vi "Boiler Controller.vi"(8 "error in":errorcluster, 9 "Controller Configuration":T1, 10 "Notifiers":T2, 11 "Message Queues":T3) -> (0 "error out":errorcluster)   [LabVIEW 2014, in "Controller.lvlib"]
uses:
  Controller.lvlib
  support/Message Queue/All Message Queues.ctl
  support/Message Queue/Message Cluster.ctl
  support/Notifiers/Notifiers.ctl
  Controller Configuration.ctl
  controls/MHL UI Data.ctl
  controls/MHL Status.ctl
  support/Boiler System Globals.vi
  <vilib>/Utility/error.llb/Error Cluster From Error Code.vi
  <vilib>/ErrorRing/Error Ring.xnode
  support/Message Queue/Message Queue.lvlib
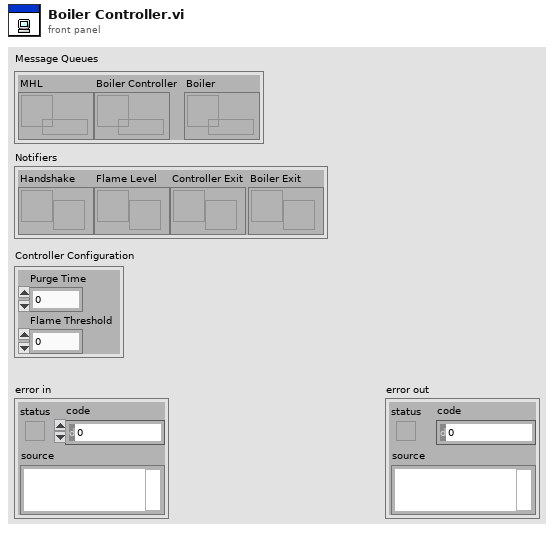
[diagram p1: front panel]
types:
  T1 = typedef "Controller.lvlib/Controller Configuration.ctl" = cluster{"Purge Time":u32, "Flame Threshold":u32}
  T2 = typedef "Notifiers.ctl" = cluster{"Handshake":refnum<notifier>, "Flame Level":refnum<notifier>, "Controller Exit":refnum<notifier>, "Boiler Exit":refnum<notifier>}
  T3 = typedef "Message Queue.lvlib/All Message Queues.ctl" = cluster{"MHL":refnum<queue>, "Boiler Controller":refnum<queue>, "Boiler":refnum<queue>}
  T4 = enum16{"open", "replace", "create", "open or create", "replace or create", "replace or create with confirmation"}
  T5 = typedef "MHL Status.ctl" = enum16{"Lockout", "Ready", "Pre-Purge", "Pre-Purge Complete", "Pilot On", "Boiler Running", "Shutdown", "Purge"}
  T6 = typedef "MHL UI Data.ctl" = cluster{"Status":string, "Fuel Control Valve":u32, "Primary Fan":bool, "Pilot Gas Valve":bool, "Pilot":bool, "Forced Draft Fan":bool, "MHL Status":T5}
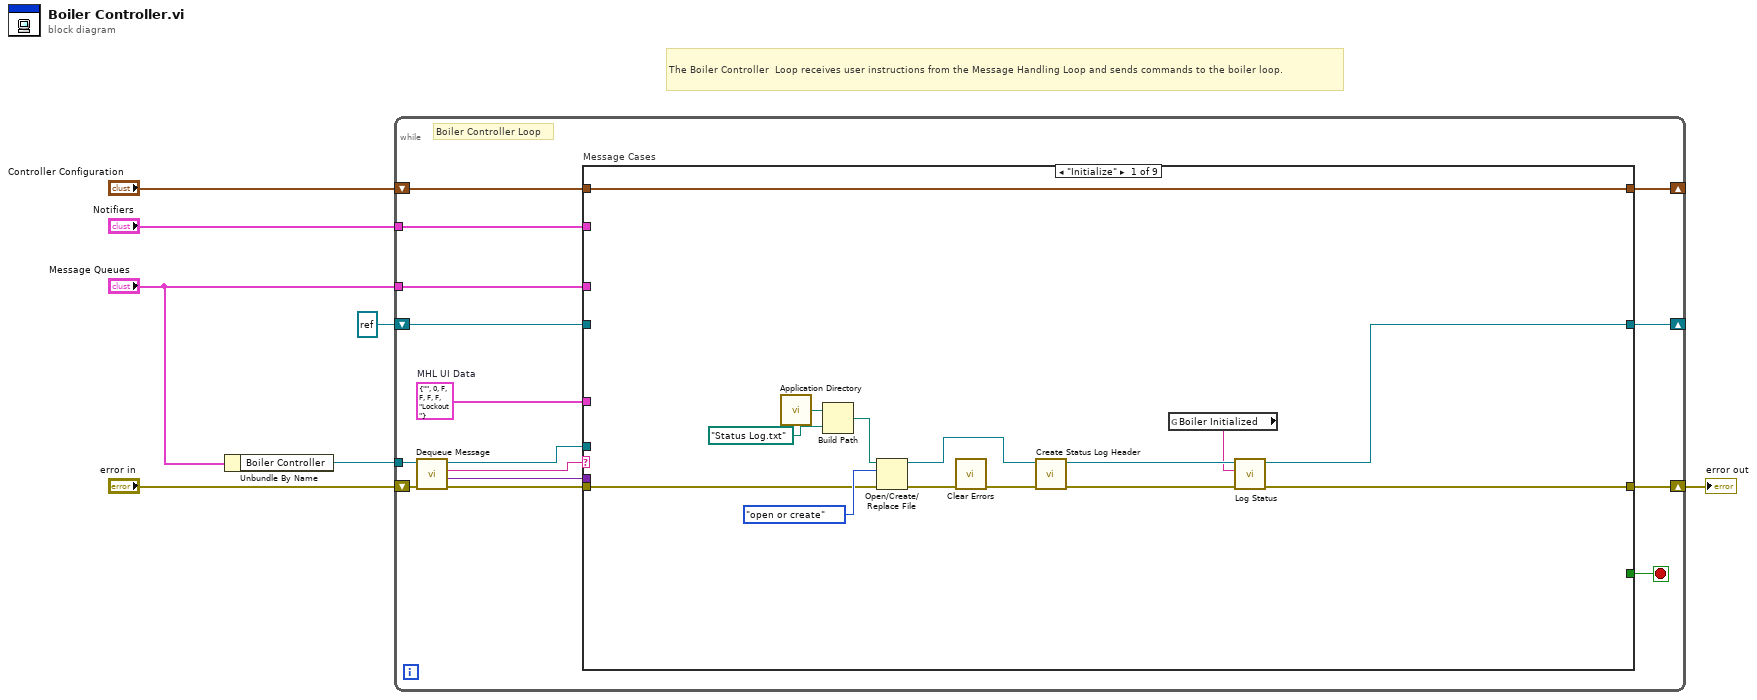
[diagram p0: block diagram]
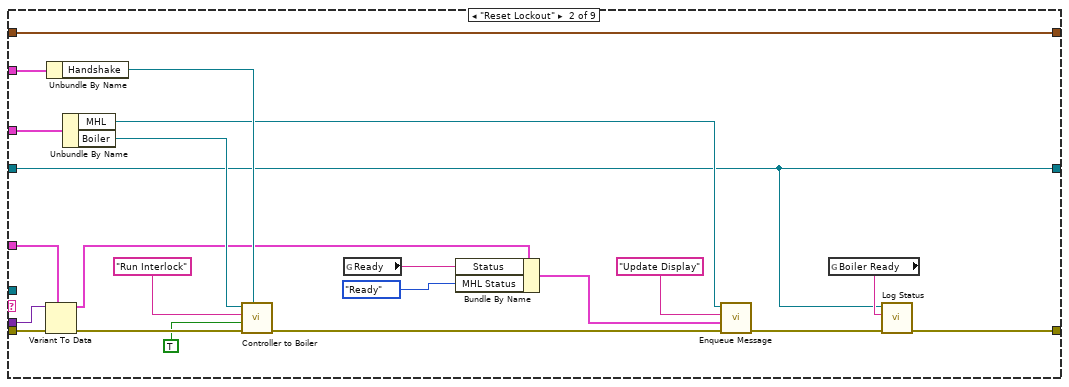
[diagram p2: hidden frame]
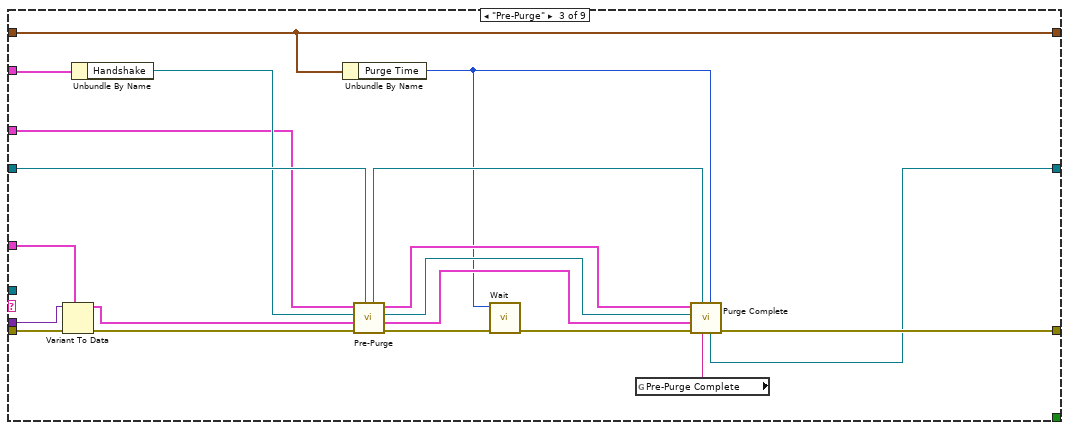
[diagram p3: hidden frame]
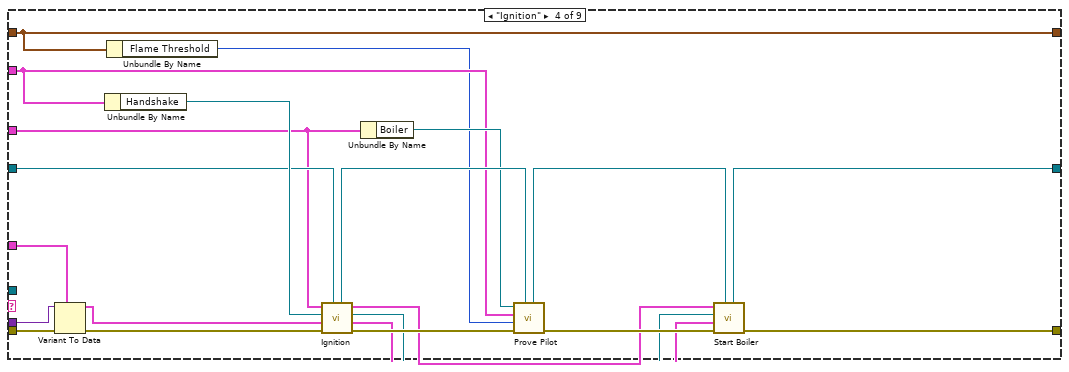
[diagram p4: hidden frame]
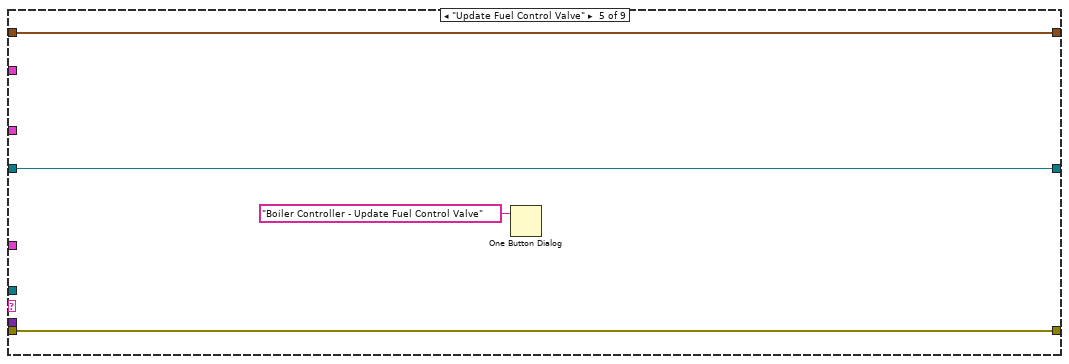
[diagram p5: hidden frame]
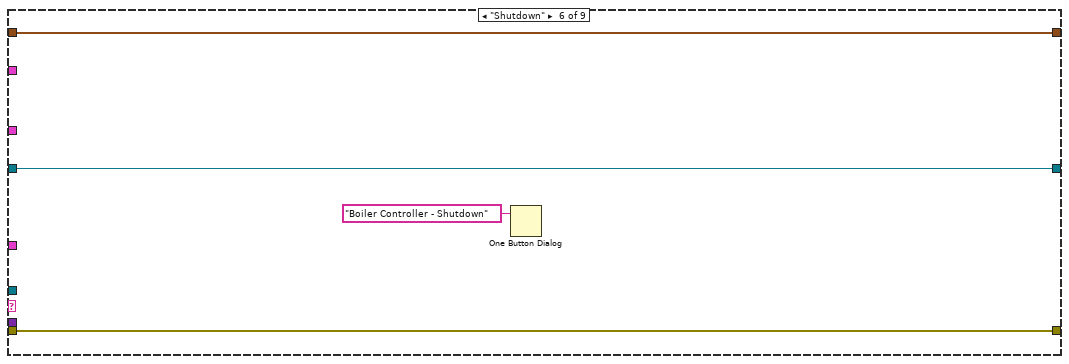
[diagram p6: hidden frame]
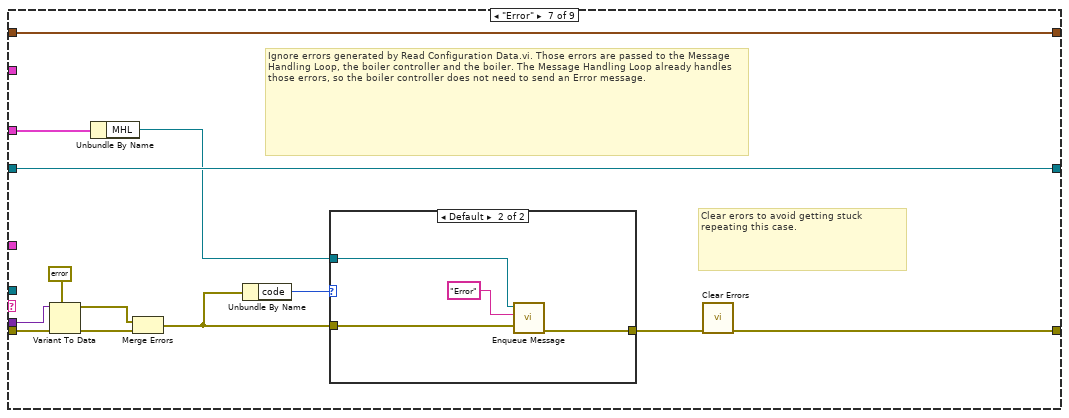
[diagram p7: hidden frame]
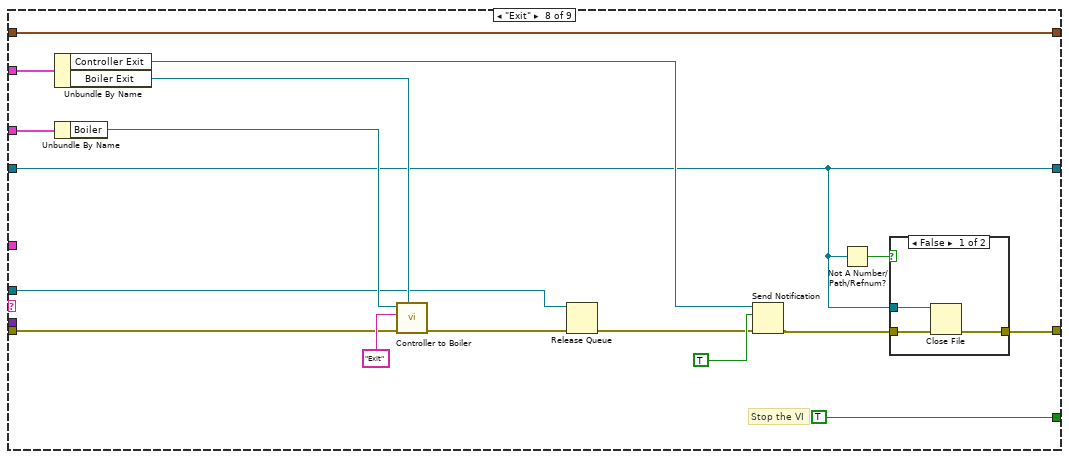
[diagram p9: hidden frame]
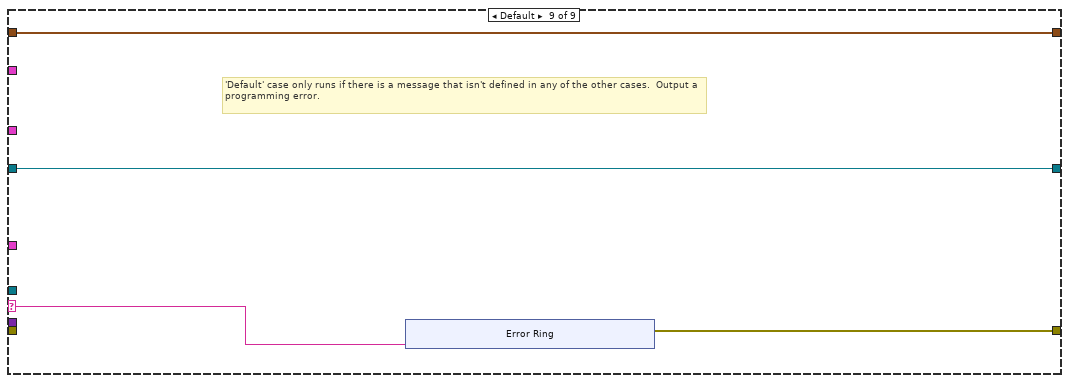
[diagram p11: hidden frame]
diagram:
  # "The Boiler Controller  Loop receives user instructions from the Message Handling Loop and sends commands to the boiler loop."
  n1 = Unbundle By Name("Message Queues") -> ("Boiler Controller"=w5:refnum<queue>)
  n2 = while {
    tunnel: w5 -> [w16]
    shift-right: [w15] -> w7
    shift-left: "error in" -> [w21]
    tunnel: "Message Queues" -> [w14]
    tunnel: "Notifiers" -> [w13]
    shift-right: [w12] -> _
    shift-left: refnum<file> refnum ("Log File Refnum out") -> [w11]
    shift-right: [w9] -> _
    shift-left: "Controller Configuration" -> [w8]
    stop <- w22 stop-if-true
    w10 = T6 {"Status"="", "Fuel Control Valve"=0, "Primary Fan"=FALSE, "Pilot Gas Valve"=FALSE, "Pilot"=FALSE, "Forced Draft Fan"=FALSE, "MHL Status"=enum."Lockout"}  # MHL UI Data
    # "Boiler Controller Loop"
    n3 = call "Dequeue Message.vi"("error in (no error)"=w21, "Message Queue"=w16) -> ("error out"=w20:errorcluster, "Message Data"=w18:variant, "Message"=w19:string, "dup Message Queue"=w17:refnum<queue>)  [unwired: 6 in]
    n4 = case "Message Cases" shown="\"Initialize\"" w19 {
      selector: w19 -> [_ _ _ _ _ _ _ _ w149]
      tunnel: w17 -> [_ _ _ _ _ _ _ w135 _]
      tunnel: w20 -> [w26 w58 w78 w99 w103 w107 w119 w134 _]
      tunnel: [w27 w54 w66 w79 w103 w107 w110 w127 w150] -> w15
      tunnel: [_ _ _ _ _ _ _ TRUE _] -> w22
      tunnel: w18 -> [_ w53 w76 w95 _ _ w117 _ _]
      tunnel: w14 -> [_ w51 w70 w89 _ _ w120 w132 _]
      tunnel: w13 -> [_ w49 w73 w87 _ _ _ w131 _]
      tunnel: [w25 w39 w64 w80 w101 w105 w114 w126 w148] -> w12
      tunnel: w11 -> [_ w39 w72 w91 w101 w105 w114 w126 w148]
      tunnel: w10 -> [_ w52 w75 w94 _ _ _ _ _]
      tunnel: w8 -> [w24 w37 w68 w86 w100 w104 w113 w130 w147]
      tunnel: [w24 w37 w68 w86 w100 w104 w113 w130 w147] -> w9
      frame "Initialize" {
        n5 = call <vilib>:"Application Directory.vi"() -> ("Application Directory"=w29:path)
        n6 = Build Path(base path=w29, name or relative path=path "Status Log.txt") -> (appended path=w33:path)
        n7 = Open/Create/Replace File(file path (use dialog)=w33, error in=w26, operation (0:open)=T4."open or create") -> (refnum out=w30:refnum<file>, error out=w31:errorcluster)  [unwired: 3 in, 1 out]
        n8 = call <vilib>:"Clear Errors.vi"("error in (no error)"=w31) -> ("error out"=w23:errorcluster)  [unwired: 5 in, 1 out]
        n9 = call "Create Status Log Header.vi"("error in"=w23, "Log File Refnum in"=w30) -> ("error out"=w36:errorcluster, "Log File Refnum out"=w35:refnum<file>)  [unwired: 8 in]
        n10 = global read "Boiler System Globals.vi" "Boiler Initialized"() -> (w34:string)
        n11 = call "Log Status.vi"("error in"=w36, "Event String"=w34, "Log File Refnum In"=w35) -> ("error out"=w27:errorcluster, "Log File Refnum Out"=w25:refnum<file>)  [unwired: 7 in]
      }
      frame "Reset Lockout" {
        n12 = Variant To Data(error in=w58, type=w52, Variant=w53) -> (data=w45:T6, error out=w57:errorcluster)
        n13 = Unbundle By Name(w49) -> ("Handshake"=w48:refnum<notifier>)
        n14 = Unbundle By Name(w51) -> ("MHL"=w41:refnum<queue>, "Boiler"=w50:refnum<queue>)
        n15 = call "Controller to Boiler.vi"("Notifier"=w48, "error in"=w57, "Message Data"=TRUE, "Message"="Run Interlock", "Boiler Queue in"=w50) -> ("error out"=w56:errorcluster)  [unwired: 4 in, 2 out]
        n16 = global read "Boiler System Globals.vi" "Ready"() -> (w44:string)
        n17 = Bundle By Name(cluster=w45, "Status"=w44, "MHL Status"=MHL_Status."Ready") -> (w43:T6)
        n18 = call "Enqueue Message.vi"("error in (no error)"=w56, "Message Data"=w43, "Message"="Update Display", "Message Queue"=w41) -> ("error out"=w55:errorcluster)  [unwired: 6 in, 1 out]
        n19 = global read "Boiler System Globals.vi" "Boiler Ready"() -> (w40:string)
        n20 = call "Log Status.vi"("error in"=w55, "Event String"=w40, "Log File Refnum In"=w39) -> ("error out"=w54:errorcluster)  [unwired: 7 in, 1 out]
      }
      frame "Pre-Purge" {
        n21 = Variant To Data(error in=w78, type=w75, Variant=w76) -> (data=w74:T6, error out=w77:errorcluster)
        n22 = Unbundle By Name(w73) -> ("Handshake"=w71:refnum<notifier>)
        n23 = Unbundle By Name(w68) -> ("Purge Time"=w60:u32)
        n24 = call "Pre-Purge.vi"("Log File Refnum in"=w72, "error in"=w77, "UI Data in"=w74, "Handshake Notifier in"=w71, "Message Queues in"=w70) -> ("error out"=w69:errorcluster, "UI Data out"=w63:T6, "Handshake Notifier out"=w62:refnum<notifier>, "Message Queues out"=w61:T3, "Log File Refnum out"=w65:refnum<file>)  [unwired: 2 in]
        n25 = call "Wait.vi"("error in"=w69, "Purge Time (s)"=w60) -> ("error out"=w67:errorcluster)  [unwired: 9 in]
        n26 = global read "Boiler System Globals.vi" "Pre-Purge Complete"() -> (w59:string)
        n27 = call "Purge Complete.vi"("Purge Time"=w60, "Status"=w59, "Log File Refnum in"=w65, "error in"=w67, "UI Data in"=w63, "Handshake Notifier in"=w62, "Message Queues in"=w61) -> ("error out"=w66:errorcluster, "Log File Refnum out"=w64:refnum<file>)  [unwired: 3 out]
      }
      frame "Ignition" {
        n28 = Variant To Data(error in=w99, type=w94, Variant=w95) -> (data=w93:T6, error out=w98:errorcluster)
        n29 = Unbundle By Name(w87) -> ("Handshake"=w92:refnum<notifier>)
        n30 = Unbundle By Name(w86) -> ("Flame Threshold"=w85:u32)
        n31 = call "Ignition.vi"("Log File Refnum in"=w91, "error in"=w98, "UI Data in"=w93, "Handshake Notifier in"=w92, "Message Queues in"=w89) -> ("error out"=w97:errorcluster, "UI Data out"=w84:T6, "Handshake Notifier out"=w83:refnum<notifier>, "Message Queues out"=w82:T3, "Log File Refnum out"=w90:refnum<file>)  [unwired: 2 in]
        n32 = Unbundle By Name(w89) -> ("Boiler"=w88:refnum<queue>)
        n33 = call "Prove Pilot.vi"("Log File Refnum in"=w90, "error in"=w97, "Flame Threshold"=w85, "Notifiers in"=w87, "Boiler Queue in"=w88) -> ("error out"=w96:errorcluster, "Log File Refnum out"=w81:refnum<file>)  [unwired: 3 in, 2 out]
        n34 = call "Start Boiler.vi"("Log File Refnum in"=w81, "error in"=w96, "UI Data in"=w84, "Handshake Notifier in"=w83, "Message Queues in"=w82) -> ("error out"=w79:errorcluster, "Log File Refnum out"=w80:refnum<file>)  [unwired: 2 in, 3 out]
      }
      frame "Update Fuel Control Valve" {
        n35 = One Button Dialog(message="Boiler Controller - Update Fuel Control Valve") -> ()  [unwired: 1 in, 1 out]
      }
      frame "Shutdown" {
        n36 = One Button Dialog(message="Boiler Controller - Shutdown") -> ()  [unwired: 1 in, 1 out]
      }
      frame "Error" {
        # "Ignore errors generated by Read Configuration Data.vi. Those errors are passed to the Message Handling Loop, the boiler controller and the boiler. The Message Handling Loop already handles those errors, so the boiler controller does not need to send an Error message."
        # "Clear erors to avoid getting stuck repeating this case."
        n37 = Variant To Data(error in=w119, type=errorcluster {"status"=FALSE, "code"=0, "source"=""} ("error out"), Variant=w117) -> (data=w115:errorcluster, error out=w116:errorcluster)
        n38 = Unbundle By Name(w120) -> ("MHL"=w109:refnum<queue>)
        n39 = Merge Errors(w115, w116) -> (w108:errorcluster)
        n40 = Unbundle By Name(w108) -> ("code"=w111:i32)
        n41 = case shown="Default" w111 {
          tunnel: w109 -> [_ w124]
          tunnel: [w121 w123] -> w112
          tunnel: w108 -> [w121 w122]
          frame 5000..5002 {
          }
          frame Default {
            n42 = call "Enqueue Message.vi"("Message Data"=w122, "Message"="Error", "Message Queue"=w124) -> ("error out"=w123:errorcluster)  [unwired: 7 in, 1 out]
          }
        }
        n43 = call <vilib>:"Clear Errors.vi"("error in (no error)"=w112) -> ("error out"=w110:errorcluster)  [unwired: 5 in, 1 out]
      }
      frame "Exit" {
        # "Stop the VI"
        n44 = Unbundle By Name(w131) -> ("Controller Exit"=w137:refnum<notifier>, "Boiler Exit"=w139:refnum<notifier>)
        n45 = Unbundle By Name(w132) -> ("Boiler"=w136:refnum<queue>)
        n46 = call "Controller to Boiler.vi"("Notifier"=w139, "error in"=w134, "Message"="Exit", "Boiler Queue in"=w136) -> ("error out"=w142:errorcluster)  [unwired: 5 in, 2 out]
        n47 = Release Queue(queue=w135, error in (no error)=w142) -> (error out=w138:errorcluster)  [unwired: 1 in, 2 out]
        n48 = Send Notification(notification=TRUE, notifier=w137, error in (no error)=w138) -> (error out=w128:errorcluster)  [unwired: 1 out]
        n49 = Not A Number/Path/Refnum?(number/path/refnum=w126) -> (NaN/Path/Refnum?=w129:bool)
        n50 = case shown="False" w129 {
          tunnel: [w144 w146] -> w127
          tunnel: w128 -> [w145 w146]
          tunnel: w126 -> [w143 _]
          frame False {
            n51 = Close File(refnum=w143, error in=w145) -> (error out=w144:errorcluster)  [unwired: 1 out]
          }
          frame True {
          }
        }
      }
      frame Default {
        # "'Default' case only runs if there is a message that isn't defined in any of the other cases.  Output a programming error."
        n52 = xnode "Error Ring"("parameter 0"=w149) -> ("error out"=w150:errorcluster)
      }
    }
  }
  "error out" <- w7
